vi "Set Version Info.vi"(6 "Description":string, 7 "Builder Configuration":T1, 8 "error in (no error)":errorcluster, 9 "Build Spec Version":T2, 10 "Name":string, 11 "NI_AB_API_PPL in":refnum<class "NI_AB_API_PPL.lvclass">) -> (0 "error out":errorcluster, 3 "NI_AB_API_PPL out":refnum<class "NI_AB_API_PPL.lvclass">)   [LabVIEW 2019]
uses:
  <vilib>/AppBuilder/AB_API/PPL/NI_AB_API_PPL.lvclass
  <vilib>/AppBuilder/AB_API/common/AB_API Version Number.ctl
  <vilib>/AppBuilder/AB_API/common/AB_API Version Information.ctl
  Builder/Builder Configuration.ctl
  Builder/Builder.lvclass
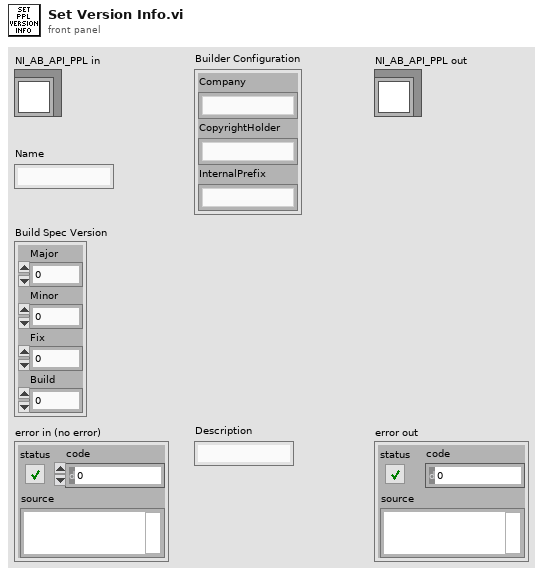
[diagram p1: front panel]
types:
  T1 = typedef "Builder.lvclass/Builder Configuration.ctl" = cluster{"Company":string, "CopyrightHolder":string, "InternalPrefix":string}
  T2 = typedef "AB_API Version Number.ctl" = cluster{"Major":u16, "Minor":u16, "Fix":u16, "Build":u16}
  T3 = typedef "AB_API Version Information.ctl" = cluster{"Product name":string, "Legal copyright":string, "Company name":string, "Internal name":string, "File description":string}
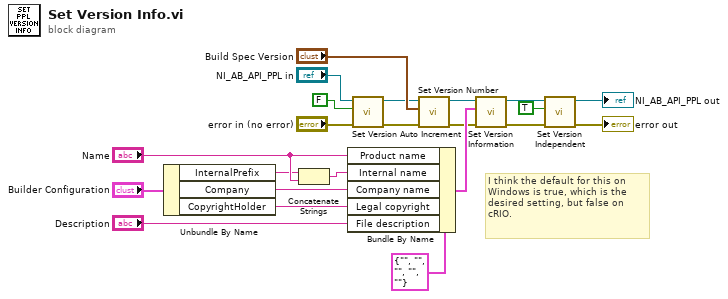
[diagram p0: block diagram]
diagram:
  # "I think the default for this on Windows is true, which is the desired setting, but false on cRIO."
  n1 = Unbundle By Name("Builder Configuration") -> ("InternalPrefix"=w2:string, "Company"=w4:string, "CopyrightHolder"=w3:string)
  n2 = Concatenate Strings(w2, "Name") -> (w11:string)
  n3 = Bundle By Name(cluster=T3 {"Product name"="", "Legal copyright"="", "Company name"="", "Internal name"="", "File description"=""} ("Version Information"), "Product name"="Name", "Internal name"=w11, "Company name"=w4, "Legal copyright"=w3, "File description"="Description") -> (w21:T3)
  n4 = call-dynamic "Set Version Auto Increment.vi"("error in (no error)"="error in (no error)", "Auto Increment Version"=FALSE, "NI_AB_API_PPL in"="NI_AB_API_PPL in") -> ("error out"=w13:errorcluster, "NI_AB_API_PPL out"=w14:refnum<class "NI_AB_API_PPL.lvclass">)  [unwired: 7 in]
  n5 = call-dynamic "Set Version Number.vi"("error in (no error)"=w13, "Version number"="Build Spec Version", "PPL in"=w14) -> ("error out"=w20:errorcluster, "PPL out"=w19:refnum<class "NI_AB_API_PPL.lvclass">)  [unwired: 7 in]
  n6 = call-dynamic "Set Version Information.vi"("error in (no error)"=w20, "Version Information"=w21, "PPL in"=w19) -> ("error out"=w8:errorcluster, "PPL out"=w10:refnum<class "NI_AB_API_PPL.lvclass">)  [unwired: 7 in]
  n7 = call-dynamic "Set Version Independent.vi"("error in (no error)"=w8, "versionIndependent"=TRUE, "NI_AB_API_PPL in"=w10) -> ("error out"=→"error out":errorcluster, "NI_AB_API_PPL out"=→"NI_AB_API_PPL out":refnum<class "NI_AB_API_PPL.lvclass">)  [unwired: 7 in]
